vi "Decrypt.vi"(11 "Input":string) -> (3 "Output":string)   [LabVIEW 2013, in "main.lvlib"]
uses:
  main.lvlib
  Controls/Enum Variables.ctl
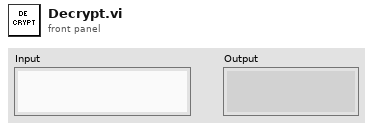
[diagram p1: front panel]
types:
  T1 = typedef "main.lvlib/Enum Variables.ctl" = enum16{"SetAcqFilter", "GetAcqFilter", "Set Filter", "Get Filter", "Set Height", "Get Height", "Set Recorded Height", "Get Recorded Height", "Set Blue Pressure", "Get Blue Pressure", "Set Red Pressure", "Get Red Pressure", "Init", "Reset Pressure", "Set Red Cursors", "Get Red Cursors", "Set Blue Cursors", "Get Blue Cursors", "Set Language", "Get Language", "Set Active Graphs", "Get ActiveGraphs", "Set Method", "Get Method", "Set Encryption", "Get Encryption", "Set ExcelVersion", "Get ExcelVersion", "Set DICOM Avail", "Get DICOM Avail", "Set DICOM Encode", "Get DICOM Encode", "Set JournalExport", "Get JournalExport", "Set Sequence", "Get Sequence", "Set DAQ Connected", "Get DAQ Connected", "Set Current Graph", "Get Current Graph", "Set General Settings", "Get Hyphenation", "Set Arm Calc Method", "Get Arm Calc Method", "Set Dicom Tags", "Get Dicom Tags", "Set BT Serial", "Get BT Serial", "Set BT Accepted Serials", "Get BT Accepted Serials", "Get BT License", "Set BT License"}
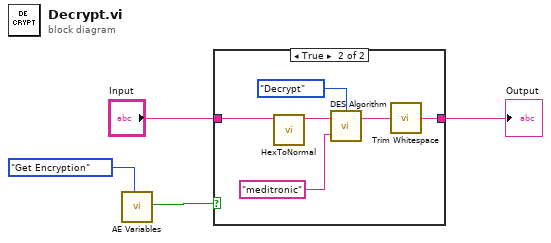
[diagram p0: block diagram]
diagram:
  n1 = call "AE Variables.vi"("Action"=Enum_Variables."Get Encryption") -> ("BooleanOut"=w1:bool)  [unwired: 11 in, 7 out]
  n2 = case shown="True" w1 {
    tunnel: [w5 w7] -> w4
    tunnel: "Input" -> [w5 w8]
    frame False {
    }
    frame True {
      n3 = call "HexToNormal.vi"("String in"=w8) -> ("String Out"=w10:string)  [unwired: 10 in]
      n4 = call <userlib>:"DES Algorithm.vi"("56 Bit Key (7 Bytes)"="meditronic", "Input"=w10, "Mode"=enum16{"Encrypt", "Decrypt"}."Decrypt") -> ("Output"=w6:string)  [unwired: 2 out]
      n5 = call <vilib>:"Trim Whitespace.vi"("string"=w6) -> ("trimmed string"=w7:string)  [unwired: 1 in]
    }
  }
  "Output" <- w4
